vi "Load Reference.vi"(8 "error in (no error)":errorcluster, 10 "Reference":refnum<vi>, 11 "ColorSelector in":refnum<class "ColorSelector.lvclass">) -> (0 "error out":errorcluster, 3 "ColorSelector out":refnum<class "ColorSelector.lvclass">)   [LabVIEW 2020, in "ColorSelector.lvclass"]
doc: "The <b>Load Reference VI</b> is a dynamic dispatch VI that must be overwritten in every QControl Class and must <b>Call Parent Method</b>. This recursively loads the reference of the control to the data space for the Control Class up the inheritance hierarchy (class hierarchy). These references must be loaded in this way to use all of the built-in properties.\n\nThe reference input is the reference type needed for the control but is coerced to Generic. It should be cast back to the correct type before bundling into the class private data. The pre-casted \"Generic\" reference is wired as input to the <b>Call Parent Method</b>.\n<b> </b> <b> </b>\n©2017 Q Software Innovations, LLC (QSI)\nwritten by Quentin Alldredge\nproduced in LabVIEW 2015\n\nsupport@qsoftwareinnovations.com\nwww.qsoftwareinnovations.com\n\nAll rights reserved.\n\nRedistribution and use in source and binary forms, with or without modification, are permitted provided that the following conditions are met:\n\n * Redistributions of source code must retain the above copyright notice, this list of conditions and the following disclaimer.\n * Redistributions in binary form must reproduce the above copyright notice, this list of conditions and the following disclaimer in the documentation and/or other materials provided with the distribution.\n * Neither the name of Q Software Innovations, LLC. nor the names of its contributors may be used to endorse or promote products derived from this software without specific prior written permission.\n\nTHIS SOFTWARE IS PROVIDED BY THE COPYRIGHT HOLDERS AND CONTRIBUTORS \"AS IS\" AND ANY EXPRESS OR IMPLIED WARRANTIES, INCLUDING, BUT NOT LIMITED TO, THE IMPLIED WARRANTIES OF MERCHANTABILITY AND FITNESS FOR A PARTICULAR PURPOSE ARE DISCLAIMED. IN NO EVENT SHALL THE COPYRIGHT OWNER OR CONTRIBUTORS BE LIABLE FOR ANY DIRECT, INDIRECT, INCIDENTAL, SPECIAL, EXEMPLARY, OR CONSEQUENTIAL DAMAGES (INCLUDING, BUT NOT LIMITED TO, PROCUREMENT OF SUBSTITUTE GOODS OR SERVICES; LOSS OF USE, DATA, OR PROFITS; OR BUSINESS INTERRUPTION) HOWEVER CAUSED AND ON ANY THEORY OF LIABILITY, WHETHER IN CONTRACT, STRICT LIABILITY, OR TORT (INCLUDING NEGLIGENCE OR OTHERWISE) ARISING IN ANY WAY OUT OF THE USE OF THIS SOFTWARE, EVEN IF ADVISED OF THE POSSIBILITY OF SUCH DAMAGE."
uses:
  ColorSelector.lvclass
  ColorSelector.lvclass/ColorSelector.ctl
  <vilib>/QSI/QControls/QControl Classes/Cluster/Cluster.lvclass
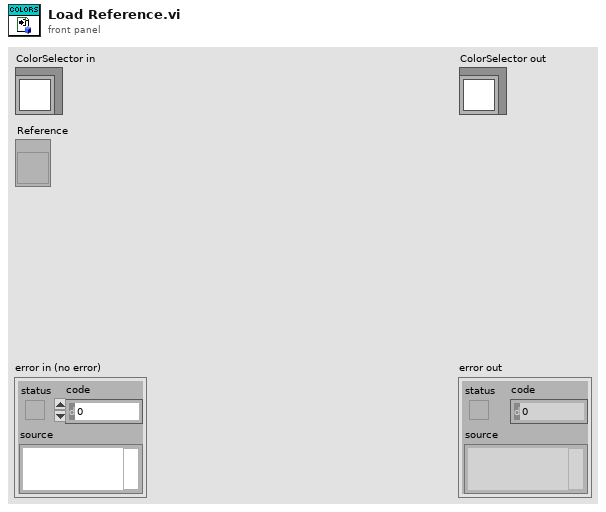
[diagram p1: front panel]
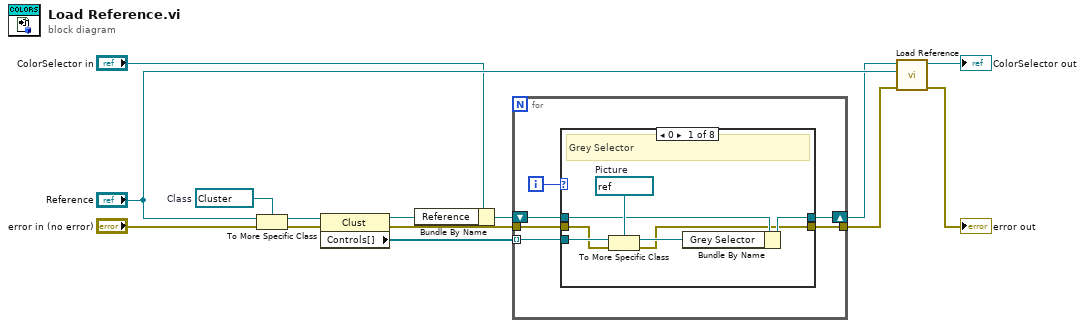
[diagram p0: block diagram]
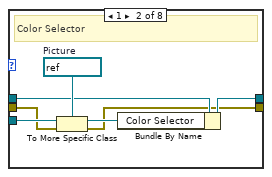
[diagram p2: hidden frame]
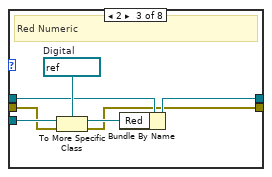
[diagram p3: hidden frame]
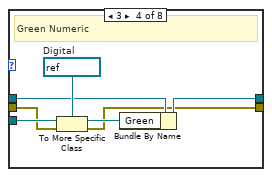
[diagram p4: hidden frame]
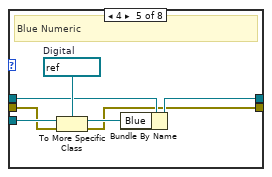
[diagram p5: hidden frame]
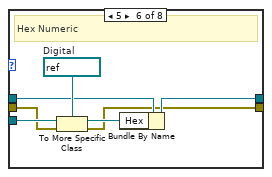
[diagram p6: hidden frame]
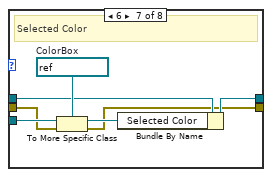
[diagram p7: hidden frame]
diagram:
  w12 = refnum<vi> refnum  # Class
  n1 = To More Specific Class(target class=w12, reference="Reference", error in="error in (no error)") -> (specific class reference=w7:refnum<vi>, error out=w14:errorcluster)
  n2 = property class="Clust"(reference=w7, error in=w14) -> (reference out=w6:refnum<vi>, error out=w2:errorcluster, "Controls[]"=w3:refnum<vi>[])
  n3 = Bundle By Name(cluster="ColorSelector in", "Reference"=w6) -> (w5:refnum<class "ColorSelector.lvclass">)
  n4 = for {
    shift-right: [w16] -> w4
    shift-left: w5 -> [w19]
    tunnel: w3 -> [w18] mode=indexing
    tunnel: w2 -> [w17]
    tunnel: [w15] -> w1
    i -> [w20]
    n5 = case shown="0" w20 {
      tunnel: w19 -> [w25 w32 w39 w46 w53 w60 w67 w70]
      tunnel: w18 -> [w27 w34 w41 w48 w55 w62 w69 _]
      tunnel: w17 -> [w23 w30 w37 w44 w51 w58 w65 w71]
      tunnel: [w21 w28 w35 w42 w49 w56 w63 w71] -> w15
      tunnel: [w22 w29 w36 w43 w50 w57 w64 w70] -> w16
      frame 0 {
        w26 = refnum<vi> refnum  # Picture
        # "Grey Selector"
        n6 = To More Specific Class(target class=w26, reference=w27, error in=w23) -> (specific class reference=w24:refnum<vi>, error out=w21:errorcluster)
        n7 = Bundle By Name(cluster=w25, "Grey Selector"=w24) -> (w22:refnum<class "ColorSelector.lvclass">)
      }
      frame 1 {
        w33 = refnum<vi> refnum  # Picture
        # "Color Selector"
        n8 = To More Specific Class(target class=w33, reference=w34, error in=w30) -> (specific class reference=w31:refnum<vi>, error out=w28:errorcluster)
        n9 = Bundle By Name(cluster=w32, "Color Selector"=w31) -> (w29:refnum<class "ColorSelector.lvclass">)
      }
      frame 2 {
        w40 = refnum<vi> refnum  # Digital
        # "Red Numeric"
        n10 = To More Specific Class(target class=w40, reference=w41, error in=w37) -> (specific class reference=w38:refnum<vi>, error out=w35:errorcluster)
        n11 = Bundle By Name(cluster=w39, "Red"=w38) -> (w36:refnum<class "ColorSelector.lvclass">)
      }
      frame 3 {
        w47 = refnum<vi> refnum  # Digital
        # "Green Numeric"
        n12 = To More Specific Class(target class=w47, reference=w48, error in=w44) -> (specific class reference=w45:refnum<vi>, error out=w42:errorcluster)
        n13 = Bundle By Name(cluster=w46, "Green"=w45) -> (w43:refnum<class "ColorSelector.lvclass">)
      }
      frame 4 {
        w54 = refnum<vi> refnum  # Digital
        # "Blue Numeric"
        n14 = To More Specific Class(target class=w54, reference=w55, error in=w51) -> (specific class reference=w52:refnum<vi>, error out=w49:errorcluster)
        n15 = Bundle By Name(cluster=w53, "Blue"=w52) -> (w50:refnum<class "ColorSelector.lvclass">)
      }
      frame 5 {
        w61 = refnum<vi> refnum  # Digital
        # "Hex Numeric"
        n16 = To More Specific Class(target class=w61, reference=w62, error in=w58) -> (specific class reference=w59:refnum<vi>, error out=w56:errorcluster)
        n17 = Bundle By Name(cluster=w60, "Hex"=w59) -> (w57:refnum<class "ColorSelector.lvclass">)
      }
      frame 6 {
        w68 = refnum<vi> refnum  # ColorBox
        # "Selected Color"
        n18 = To More Specific Class(target class=w68, reference=w69, error in=w65) -> (specific class reference=w66:refnum<vi>, error out=w63:errorcluster)
        n19 = Bundle By Name(cluster=w67, "Selected Color"=w66) -> (w64:refnum<class "ColorSelector.lvclass">)
      }
      frame Default {
        # "This Case Not Used"
      }
    }
  }
  n20 = call-parent "Load Reference.vi"("error in (no error)"=w1, "Reference"="Reference", "Cluster in"=w4) -> ("error out"=→"error out":errorcluster, "Cluster out"=→"ColorSelector out":refnum<class "ColorSelector.lvclass">)  [unwired: 7 in]
